vi "sub_Gslam_observation.vi"(8 "rf id":cluster{"x":dbl, "y":dbl, "yaw":dbl}[](array[cluster]), 9 "u":T1, 10 "xd":T1, 11 "x_true":T1) -> (0 "ud":T1, 1 "xd out":T1, 2 "z":T1, 3 "x_true out":T1)   [LabVIEW 2019]
uses:
  <vilib>/Analysis/Matrix/Datatypes/RealMatrix.ctl
  Ctrl/cmd_common.ctl
  <vilib>/ptbypt/NI_PtbyPt.lvlib
  <vilib>/Analysis/Matrix/NI_Matrix.lvlib
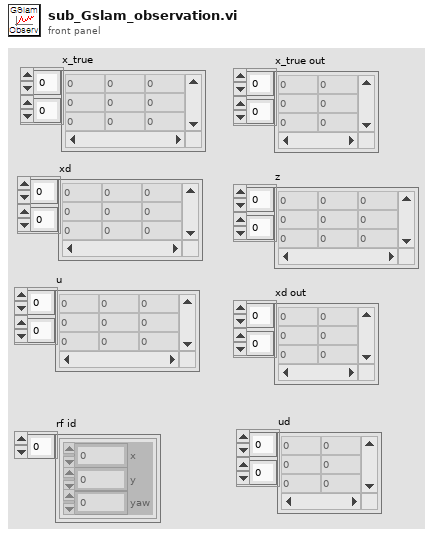
[diagram p1: front panel]
types:
  T1 = typedef "NI_Matrix.lvlib/RealMatrix.ctl" = dbl[][]
  T2 = typedef "cmd_common.ctl" = enum16{"read", "write"}
  T3 = cluster{"Q Sim":T1, "R Sim":T1, "DT":dbl, "SIM_TIME":dbl, "MAX_RANGE":dbl, "STATE_SIZE":i32, "C_SIGMA 1":dbl, "C_SIGMA 2":dbl, "C_SIGMA 3":dbl, "MAX_ITR":u32}
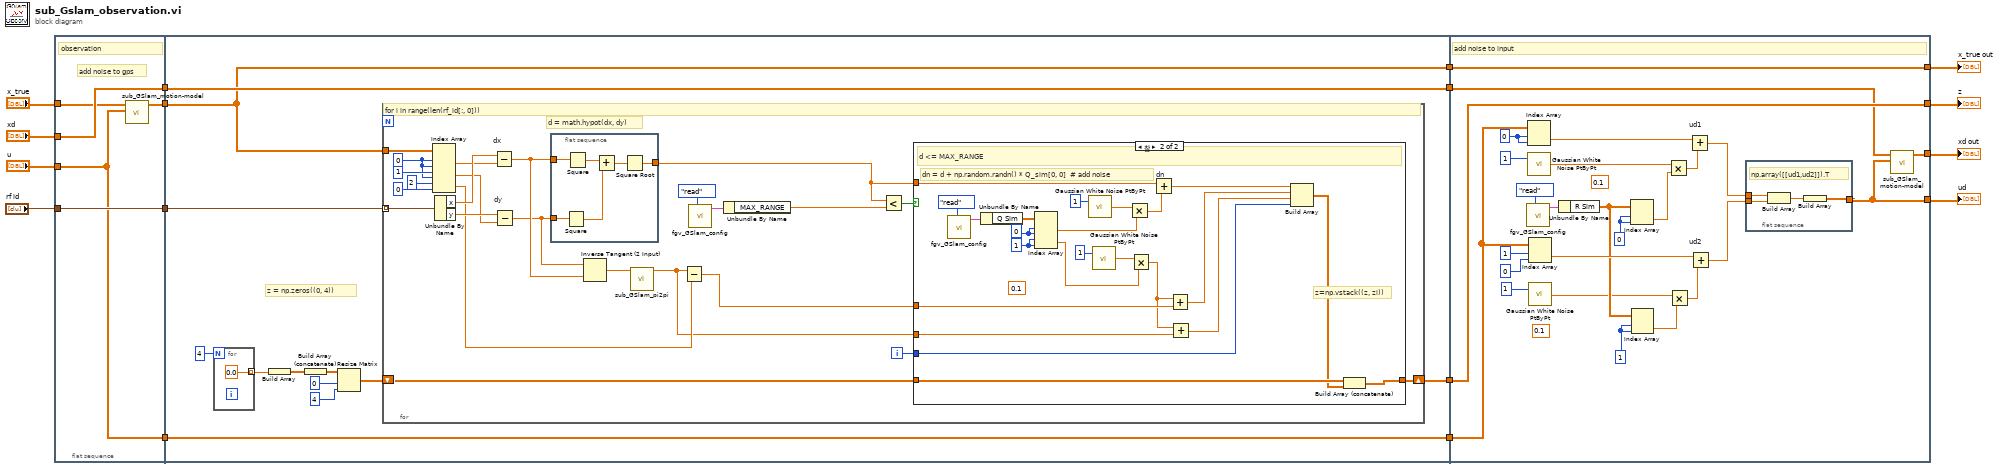
[diagram p0: block diagram]
diagram:
  n1 = flat-sequence {
    tunnel: "u" -> [w18]
    tunnel: [w21] -> w16
    tunnel: "x_true" -> [w19]
    tunnel: "rf id" -> [w21]
    tunnel: [w20] -> w15
    tunnel: [w18] -> w14
    tunnel: [w17] -> w13
    tunnel: "xd" -> [w20]
    tunnel: w16 -> [w22]
    tunnel: [w31] -> w12
    tunnel: [w33] -> w11
    tunnel: w15 -> [w32]
    tunnel: [w32] -> w10
    tunnel: [w30] -> w9
    tunnel: w14 -> [w31]
    tunnel: w13 -> [w30]
    tunnel: w12 -> [w103]
    tunnel: [w98] -> w3
    tunnel: [w97] -> w4
    tunnel: w11 -> [w99]
    tunnel: [w99] -> w5
    tunnel: w10 -> [w96]
    tunnel: w9 -> [w100]
    tunnel: [w100] -> w6
    frame #0 {
      # "add noise to gps"
      # "observation"
      n2 = call "sub_GSlam_motion-model.vi"("u"=w18, "x_true"=w19) -> ("x_true out"=w17:T1)  [unwired: 9 in]
    }
    frame #1 {
      # "z = np.zeros((0, 4))"
      n3 = for {
        N: 4 -> [_]
        tunnel: [0.0] -> w28 mode=indexing
      }
      n4 = Build Array(w28) -> (w27:dbl[][])
      n5 = Build Array (concatenate)(w27) -> (w26:T1)
      n6 = Resize Matrix(1:4 ("행의 개수"), 2:0 ("행의 개수"), 4:w26) -> (0:w25:T1)
      n7 = for {
        shift-right: [w53] -> w33
        shift-left: w25 -> [w54]
        tunnel: w30 -> [w52]
        tunnel: w22 -> [w48] mode=indexing
        i -> [w35]
        w57 = 0 ("인덱스 (행)")
        # "d = math.hypot(dx, dy)"
        # "for i in range(len(rf_id[:, 0]))"
        n8 = Index Array(array=w52, index (row) #1=w57, index (col) #1=w57, index (row) #2=1 ("인덱스 (행)"), index (col) #2=w57, index (row) #3=2 ("index (col)"), index (col) #3=0 ("index (col)")) -> (element #1=w46:dbl, element #2=w44:dbl, element #3=w38:dbl)
        n9 = Unbundle By Name(w48) -> ("x"=w47:dbl, "y"=w45:dbl)
        n10 = Subtract "dx"(x=w47, y=w46) -> (x-y=w43:dbl)
        n11 = Subtract "dy"(x=w45, y=w44) -> (x-y=w42:dbl)
        n12 = flat-sequence {
          tunnel: w42 -> [w64]
          tunnel: w43 -> [w63]
          tunnel: [w59] -> w51
          frame #0 {
            n13 = Square(x=w64) -> (x^2=w60:dbl)
            n14 = Square(x=w63) -> (x^2=w61:dbl)
            n15 = Add(x=w61, y=w60) -> (x+y=w62:dbl)
            n16 = Square Root(x=w62) -> (sqrt(x)=w59:dbl)
          }
        }
        n17 = Inverse Tangent (2 Input)(1:w43, 2:w42) -> (0:w41:dbl)
        n18 = call "sub_GSlam_pi2pi.vi"("angle"=w41) -> ("result"=w36:dbl)  [unwired: 10 in]
        n19 = Subtract(x=w36, y=w38) -> (x-y=w37:dbl)
        n20 = call "fgv_GSlam_config.vi"("cmd"=cmd_common."read") -> ("G cofnig out"=w50:T3)  [unwired: 10 in]
        n21 = Unbundle By Name(w50) -> ("MAX_RANGE"=w56:dbl)
        n22 = Less?(x=w51, y=w56) -> (x < y?=w55:bool)
        n23 = case shown="참" w55 {
          tunnel: w51 -> [_ w85]
          tunnel: w54 -> [w65 w82]
          tunnel: [w65 w83] -> w53
          tunnel: w37 -> [_ w73]
          tunnel: w36 -> [_ w71]
          tunnel: w35 -> [_ w68]
          frame False {
          }
          frame True {
            (unwired) 0.1
            w77 = 1 ("인덱스 (행)")
            w76 = 0 ("인덱스 (행)")
            # "dn = d + np.random.randn() * Q_sim[0, 0]  # add noise"
            # "z=np.vstack((z, zi))"
            # "d <= MAX_RANGE"
            n24 = call "fgv_GSlam_config.vi"("cmd"=cmd_common."read") -> ("G cofnig out"=w79:T3)  [unwired: 10 in]
            n25 = Unbundle By Name(w79) -> ("Q Sim"=w87:T1)
            n26 = Index Array(array=w87, index (row) #1=w76, index (col) #1=w76, index (row) #2=w77, index (col) #2=w77) -> (element #1=w78:dbl, element #2=w74:dbl)
            n27 = call <vilib>:"Gaussian White Noise PtByPt.vi"("standard deviation"=1 ("samples")) -> ("Gaussian white noise"=w67:dbl)  [unwired: 2 in]
            n28 = call <vilib>:"Gaussian White Noise PtByPt.vi"("standard deviation"=1 ("samples")) -> ("Gaussian white noise"=w66:dbl)  [unwired: 2 in]
            n29 = Multiply(x=w67, y=w78) -> (x*y=w86:dbl)
            n30 = Multiply(x=w66, y=w74) -> (x*y=w72:dbl)
            n31 = Add "dn"(x=w85, y=w86) -> (x+y=w84:dbl)
            n32 = Add(x=w72, y=w73) -> (x+y=w70:dbl)
            n33 = Add(x=w72, y=w71) -> (x+y=w69:dbl)
            n34 = Build Array(w84, w70, w69, w68) -> (w81:T1)
            n35 = Build Array (concatenate)(w82, w81) -> (w83:T1)
          }
        }
      }
    }
    frame #2 {
      (unwired) 0.1
      (unwired) 0.1
      w107 = 1 ("인덱스 (행)")
      w112 = 0 ("인덱스 (행)")
      w114 = 0 ("인덱스 (행)")
      # "add noise to input"
      n36 = call "fgv_GSlam_config.vi"("cmd"=cmd_common."read") -> ("G cofnig out"=w94:T3)  [unwired: 10 in]
      n37 = Index Array(array=w103, index (row)=w114, index (col)=w114) -> (element=w110:dbl)
      n38 = call <vilib>:"Gaussian White Noise PtByPt.vi"("standard deviation"=1 ("samples")) -> ("Gaussian white noise"=w90:dbl)  [unwired: 2 in]
      n39 = Index Array(array=w103, index (row)=1 ("인덱스 (행)"), index (col)=0 ("인덱스 (행)")) -> (element=w109:dbl)
      n40 = call <vilib>:"Gaussian White Noise PtByPt.vi"("standard deviation"=1 ("samples")) -> ("Gaussian white noise"=w89:dbl)  [unwired: 2 in]
      n41 = Unbundle By Name(w94) -> ("R Sim"=w93:T1)
      n42 = Index Array(array=w93, index (row)=w112, index (col)=w112) -> (element=w92:dbl)
      n43 = Index Array(array=w93, index (row)=w107, index (col)=w107) -> (element=w91:dbl)
      n44 = Multiply(x=w90, y=w92) -> (x*y=w111:dbl)
      n45 = Multiply(x=w89, y=w91) -> (x*y=w108:dbl)
      n46 = Add "ud1"(x=w110, y=w111) -> (x+y=w102:dbl)
      n47 = Add "ud2"(x=w109, y=w108) -> (x+y=w101:dbl)
      n48 = flat-sequence {
        tunnel: w102 -> [w118]
        tunnel: w101 -> [w117]
        tunnel: [w116] -> w97
        frame #0 {
          # "np.array([[ud1,ud2]]).T"
          n49 = Build Array(w118, w117) -> (w115:dbl[])
          n50 = Build Array(w115) -> (w116:T1)
        }
      }
      n51 = call "sub_GSlam_motion-model.vi"("u"=w97, "x_true"=w96) -> ("x_true out"=w98:T1)  [unwired: 9 in]
    }
  }
  "x_true out" <- w6
  "z" <- w5
  "ud" <- w4
  "xd out" <- w3
